vi "GetTotePos.vi"(3 "Bottom Right":cluster{"x":i16, "y":i16}, 4 "Bottom Left":cluster{"x":i16, "y":i16}, 5 "Top Right":cluster{"x":i16, "y":i16}, 6 "Top Left":cluster{"x":i16, "y":i16}) -> (0 "X Offset":dbl=-2.5, 1 "Angle":dbl, 2 "Distance":dbl=15.0)   [LabVIEW 2014]
panel:
  in  "Picking up from side?":bool
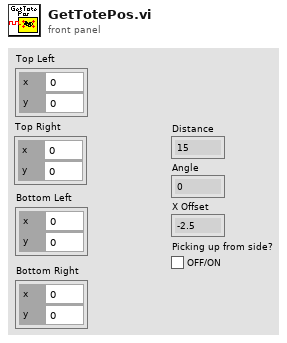
[diagram p1: front panel]
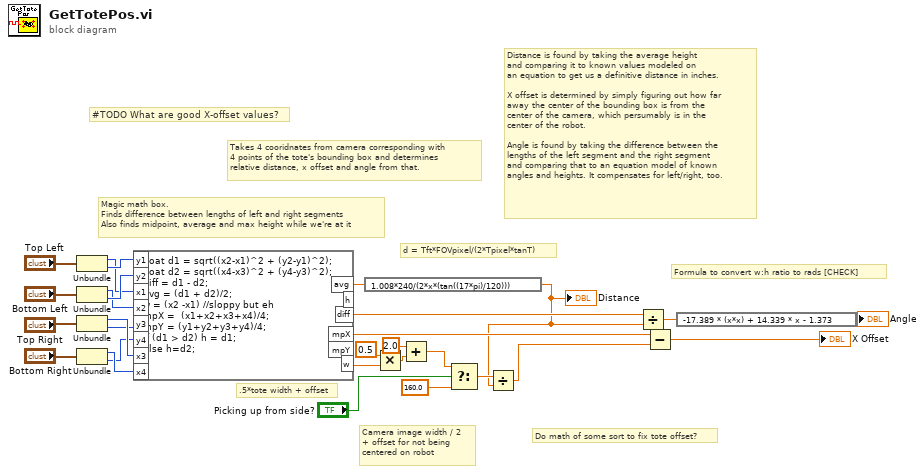
[diagram p0: block diagram]
diagram:
  # ".5*tote width + offset"
  # "#TODO What are good X-offset values?"
  # "Do math of some sort to fix tote offset?"
  # "Distance is found by taking the average height\nand comparing it to known values modeled on\nan equation to get us a definitive distance in inches.\n\nX offset is determined by simply figuring out how far\naway the center of the bounding box is from the\ncenter of the camera, which persumably is in the\ncenter of the robot.\n\nAngle is found by taking the difference between the\nlengths of the left segment and the right segment\nand comparing that to an equation model of known\nangles and heights. It compensates for left/right, too."
  # "Camera image width / 2\n+ offset for not being \ncentered on robot"
  # "Formula to convert w:h ratio to rads [CHECK]"
  # "d = Tft*FOVpixel/(2*Tpixel*tanT)"
  # "Magic math box.\nFinds difference between lengths of left and right segments\nAlso finds midpoint, average and max height while we're at it"
  # "Takes 4 cooridnates from camera corresponding with\n4 points of the tote's bounding box and determines\nrelative distance, x offset and angle from that."
  n1 = Unbundle("Top Left") -> ("x"=w24:i16, "y"=w26:i16)
  n2 = Unbundle("Bottom Left") -> ("x"=w23:i16, "y"=w25:i16)
  n3 = Unbundle("Top Right") -> ("x"=w20:i16, "y"=w17:i16)
  n4 = Unbundle("Bottom Right") -> ("x"=w19:i16, "y"=w18:i16)
  n5 = formula code="float d1 = sqrt((x2-x1)^2 + (y2-y1)^2);\nfloat d2 = sqrt((x4-x3)^2 + (y4-y3)^2);\ndiff = d1 - d2;\navg = (d1 + d2)/2;\nw = (x2 -x1) //sloppy but eh\nmpX =  (x1+x2+x3+x4)/4;\nmpY = (y1+y2+y3+y4)/4;\nif (d1 > d2) h = d1; \nelse h=d2;"("y1"=w26, "y2"=w25, "x1"=w24, "x2"=w23, "y3"=w17, "y4"=w18, "x3"=w20, "x4"=w19) -> ("diff"=w15:dbl, "mpX"=w12:dbl, "avg"=w16:dbl, "w"=w4:dbl)  [unwired: 2 out]
  n6 = expression code="1.008*240/(2*x*(tan((17*pi)/120)))"(w16) -> (w7:dbl)
  "Distance" <- w7
  n7 = Multiply(x=0.5, y=w4) -> (x*y=w3:dbl)
  n8 = Add(x=2.0, y=w3) -> (x+y=w2:dbl)
  n9 = Select(t=w2, s="Picking up from side?", f=160.0 ("y")) -> (s? t:f=w9:dbl)
  n10 = Divide(x=w9, y=w7) -> (x/y=w8:dbl)
  n11 = Divide(x=w15, y=w7) -> (x/y=w14:dbl)
  n12 = Subtract(x=w12, y=w8) -> (x-y=→"X Offset":dbl)
  n13 = expression code="-17.389 * (x*x) + 14.339 * x - 1.373"(w14) -> (→"Angle":dbl)
